vi "camara 2.1.vi"() -> ()   [LabVIEW 2010]
uses:
  <vilib>/addons/PixeLINK/Low Level Functions/CAMERA_FEATURES.llb/TDPU-CameraFeatures-PixelFormat.ctl
  <vilib>/addons/PixeLINK/Low Level Functions/ACQUISITION.llb/TDPU-Acquisition-StreamState.ctl
  <vilib>/addons/PixeLINK/Low Level Functions/CAMERA_FEATURES.llb/TDPU-CameraFeatures-FeatureFlags.ctl
  <vilib>/addons/PixeLINK/Low Level Functions/CAMERA_FEATURES.llb/TDPU-CameraFeatures-FeatureIds.ctl
panel:
  in  "Gain":dbl(slide) scale=0.0..25.0
  out "size(s)":i32
  out "Data OUT":u32[](array[numeric]) format="%x"
  out "Image":T1(plugin-control)
  out "output array":u64[][](array[numeric]) format="%x"
  in  "Exposure Time (ms)":dbl(slide) scale=0.1..2000.0
  in  "Streeam":bool
  in  "Pixel Format Requerido":T2 items=["PIXEL_FORMAT_MONO8", "PIXEL_FORMAT_MONO16", "PIXEL_FORMAT_YUV422", "PIXEL_FORMAT_BAYER8_GRBG", "PIXEL_FORMAT_BAYER16_GRBG", "PIXEL_FORMAT_RGB24", "PIXEL_FORMAT_RGB48", "PIXEL_FORMAT_BAYER8_RGGB", "PIXEL_FORMAT_BAYER8_GBRG ", "PIXEL_FORMAT_BAYER8_BGGR ", "PIXEL_FORMAT_BAYER16_RGGB ", "PIXEL_FORMAT_BAYER16_GBRG", "PIXEL_FORMAT_BAYER16_BGGR", "PIXEL_FORMAT_RGB32"]
  out "Numeric":i32
  in  "Stop App":bool
  out "Numero de Camaras":u32
  in  "Selector":u16(ring) items=["776002034"]
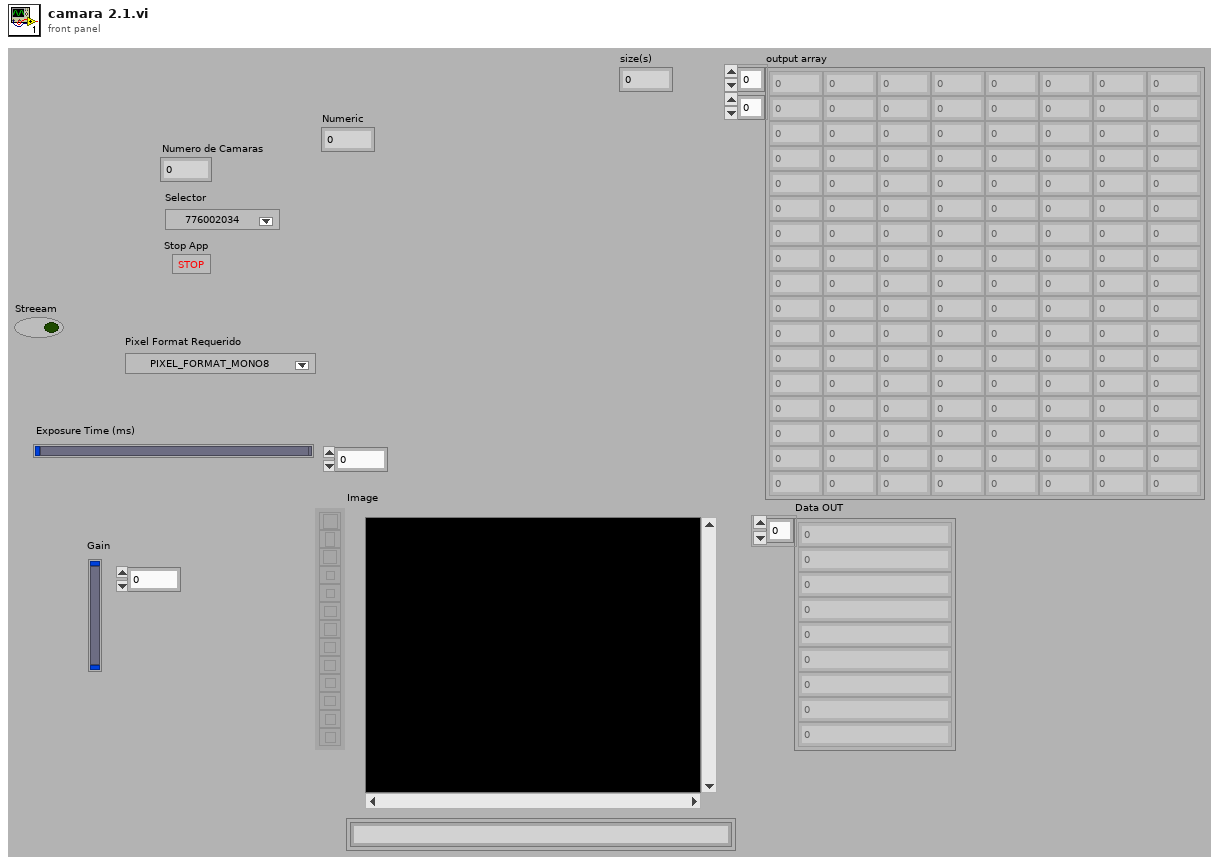
[diagram p1: front panel]
types:
  T1 = typedef "IMAQ Image.ctl" = refnum<image>
  T2 = typedef "TDPU-CameraFeatures-PixelFormat.ctl" = u16
  T3 = typedef "Image Type" = u32
  T4 = typedef "TDPU-Acquisition-StreamState.ctl" = u32
  T5 = typedef "TDPU-CameraFeatures-FeatureIds.ctl" = u32
  T6 = typedef "TDPU-CameraFeatures-FeatureFlags.ctl" = u32
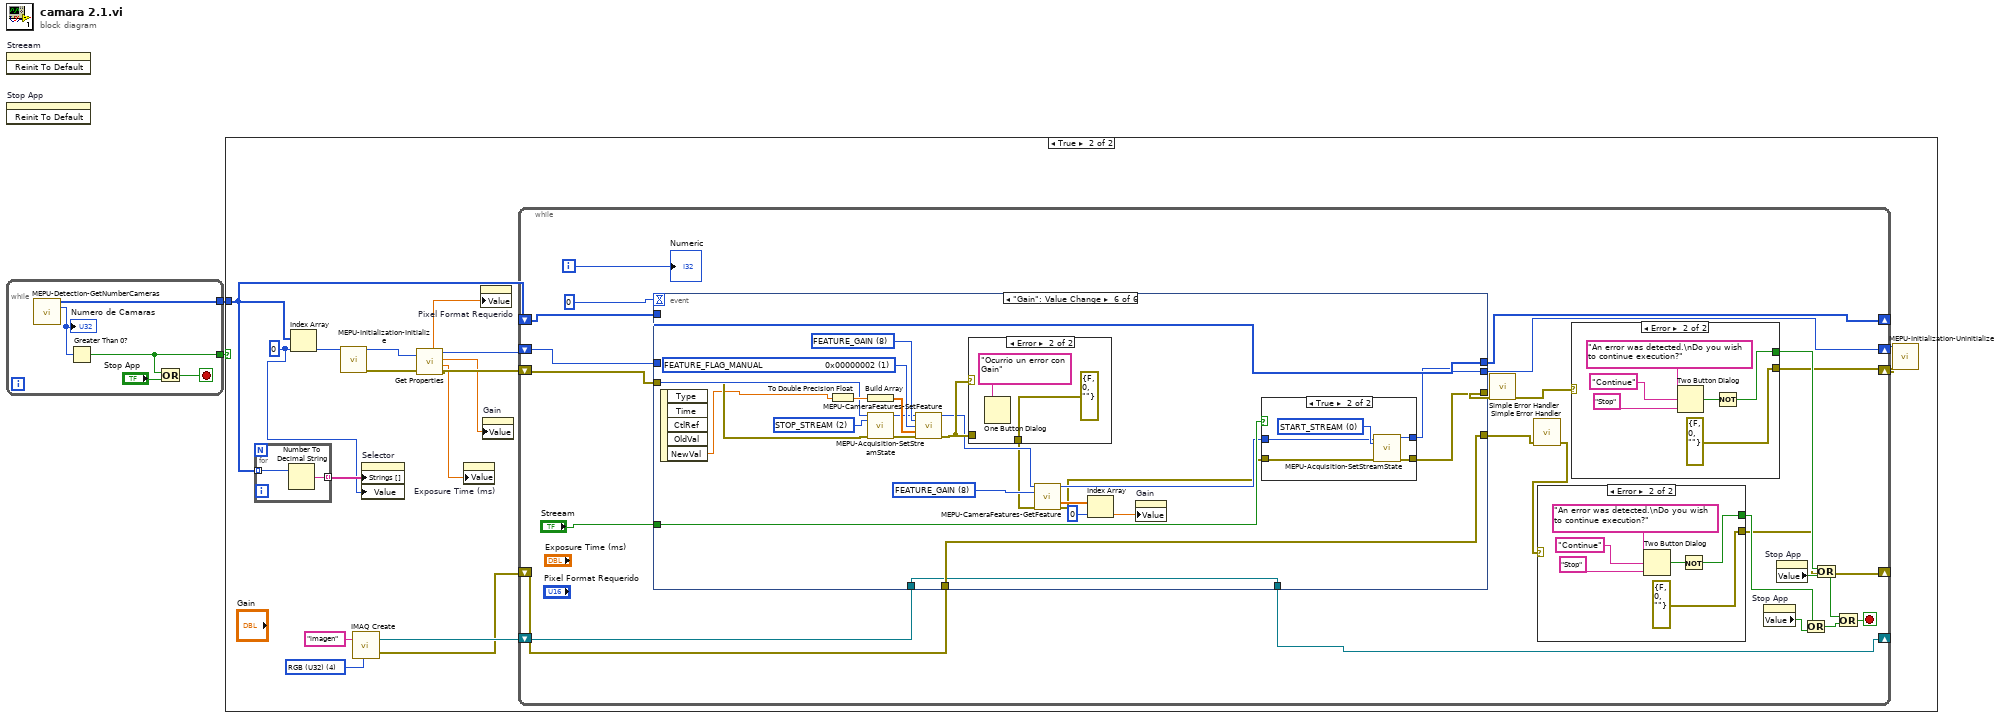
[diagram p0: block diagram]
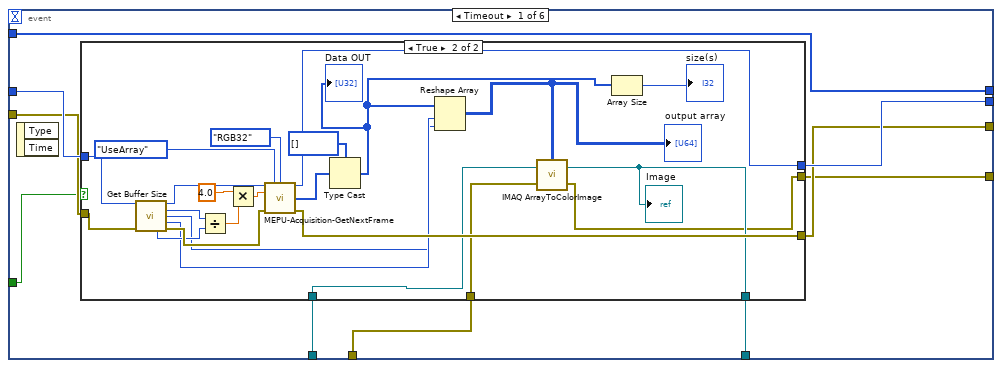
[diagram p5: hidden frame]
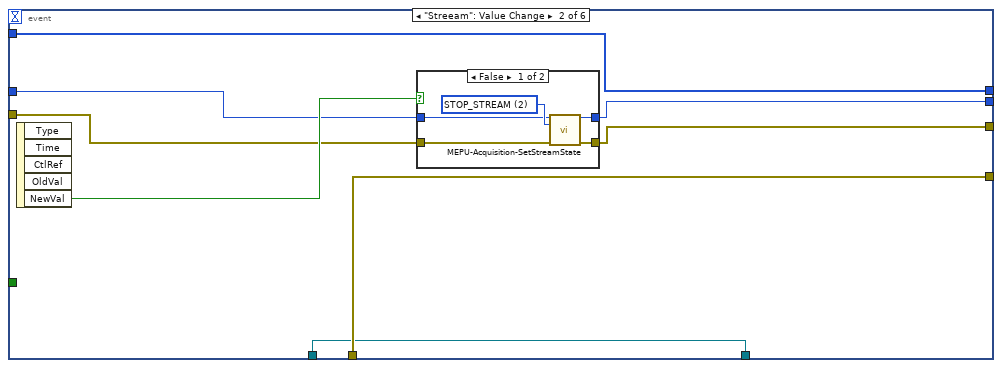
[diagram p7: hidden frame]
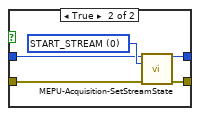
[diagram p8: hidden frame]
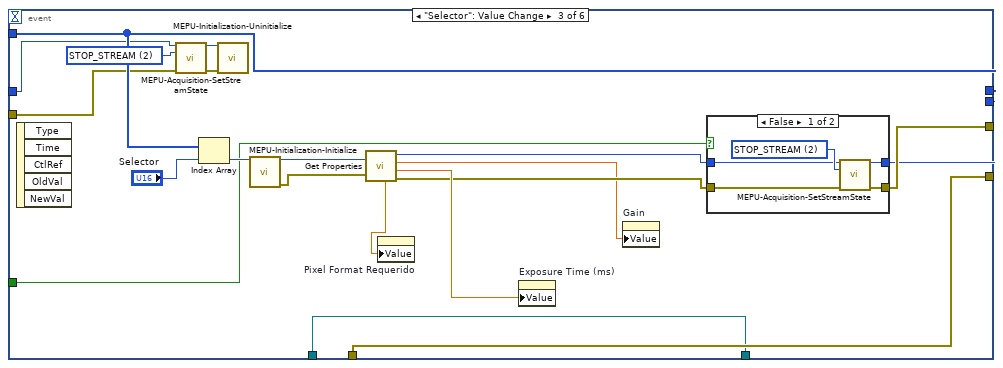
[diagram p9: hidden frame]
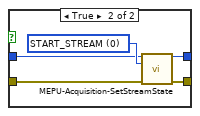
[diagram p10: hidden frame]
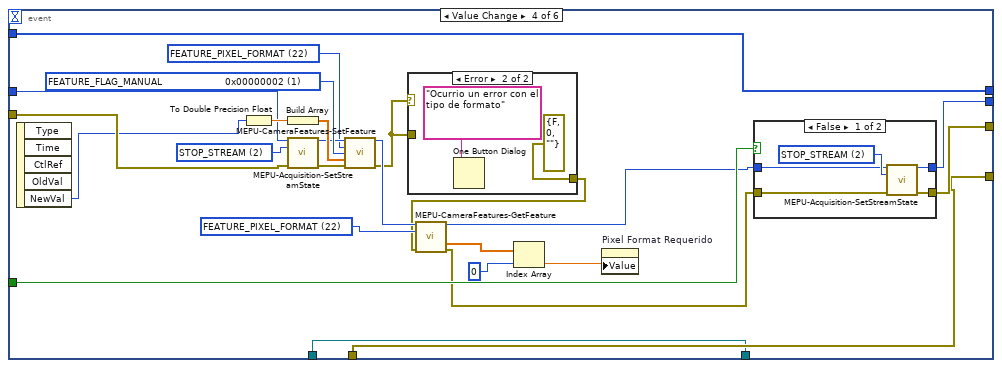
[diagram p11: hidden frame]
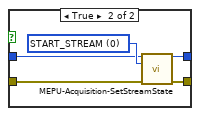
[diagram p12: hidden frame]
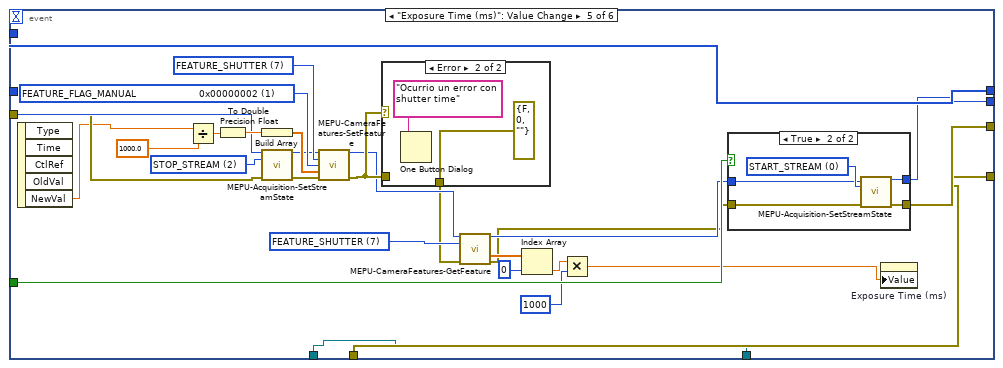
[diagram p14: hidden frame]
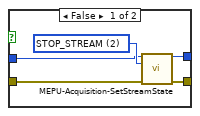
[diagram p15: hidden frame]
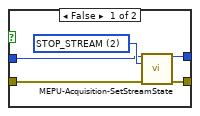
[diagram p17: hidden frame]
diagram:
  n1 = invoke on="Streeam" class="Bool (strict)" method="Reinit To Default"() -> ()  [unwired: 3 in, 3 out]
  n2 = invoke on="Stop App" class="Bool (strict)" method="Reinit To Default"() -> ()  [unwired: 3 in, 3 out]
  n3 = while {
    tunnel: [w7] -> w2
    tunnel: [w3] -> w1
    stop <- w5 stop-if-true
    n4 = call <vilib>:"MEPU-Detection-GetNumberCameras.vi"() -> ("LV_SerialNumbers OUT"=w7:u32[], "LV_NumberSerial OUT"=w4:u32)  [unwired: 13 in, 1 out]
    "Numero de Camaras" <- w4
    n5 = Greater Than 0?(x=w4) -> (x > 0?=w3:bool)
    n6 = Or(x=w3, y="Stop App") -> (x .or. y?=w5:bool)
  }
  n7 = case shown="True" w1 {
    tunnel: w2 -> [_ w21]
    frame False {
    }
    frame True {
      w15 = T3 4 items=["Grayscale (U8)", "Grayscale (I16)", "Grayscale (SGL)", "Complex (CSG)", "RGB (U32)", "HSL (U32)", "RGB (U64)", "Grayscale (U16)"] ("Image Type")
      w20 = 0
      n8 = for {
        tunnel: w21 -> [w269] mode=indexing
        tunnel: [w268] -> w23 mode=indexing
        n9 = Number To Decimal String(number=w269) -> (decimal integer string=w268:string)  [unwired: 1 in]
      }
      n10 = Index Array(array=w21, index=w20) -> (element=w22:u32)
      n11 = call <vilib>:"MEPU-Initialization-Initialize.vi"("uSerialNumber IN"=w22) -> ("phCamera OUT"=w14:u32, "Error OUT"=w13:errorcluster)  [unwired: 12 in, 1 out]
      n12 = call "IMAQ Create"("Image Name"="imagen", "Image Type"=w15) -> ("New Image"=w18:T1, "error out"=w16:errorcluster)  [unwired: 3 in]
      n13 = property on="Selector" class="Ring (strict)"("Strings []"=w23, "Value"=w20) -> ()  [unwired: 2 in, 2 out]
      n14 = call "Get Properties.vi"("phCamera IN"=w14, "Error IN"=w13) -> ("hCamera OUT"=w12:u32, "Gain OUT"=w10:dbl, "Shutter Time OUT (ms)"=w8:dbl, "Error OUT"=w11:errorcluster, "Pixel Format OUT"=w9:dbl)
      n15 = property on="Exposure Time (ms)" class="Slide (strict)"("Value"=w8) -> ()  [unwired: 2 in, 2 out]
      n16 = property on="Pixel Format Requerido" class="Ring (strict)"("Value"=w9) -> ()  [unwired: 2 in, 2 out]
      n17 = property on="Gain" class="Slide (strict)"("Value"=w10) -> ()  [unwired: 2 in, 2 out]
      n18 = while {
        shift-right: [w46] -> _
        shift-left: w21 -> [w47]
        shift-right: [w36] -> w19
        shift-left: w12 -> [w45]
        shift-right: [w41] -> _
        shift-left: w11 -> [w44]
        shift-right: [w26] -> _
        shift-left: w16 -> [w25]
        shift-right: [w24] -> _
        shift-left: w18 -> [w34]
        i -> [w40]
        stop <- w28 stop-if-true
        n19 = event shown="[5] \"Gain\": Value Change" {
          selector: _ -> [_ _ _ _ _ _]
          dyn-events: _ -> [_ _ _ _ _ _]
          timeout: 0 -> [_ _ _ _ _ _]
          tunnel: w47 -> [w73 w102 w137 w166 w208 w246]
          tunnel: [w71 w106 w128 w165 w207 w245] -> w36
          tunnel: [w68 w105 w129 w164 w206 w244] -> w37
          tunnel: [w73 w102 w137 w166 w208 w246] -> w46
          tunnel: w45 -> [w72 w108 w130 w171 w205 w243]
          tunnel: w44 -> [w70 w107 w131 w170 w204 w242]
          tunnel: "Streeam" -> [w69 _ w127 w163 w203 w241]
          tunnel: w34 -> [w67 w103 w125 w151 w189 w232]
          tunnel: w25 -> [w66 w104 w126 w162 w200 w240]
          tunnel: [w65 w104 w126 w162 w200 w240] -> w33
          tunnel: [w64 w103 w125 w151 w189 w232] -> w24
          event Timeout {
            n20 = event-data() -> ()  [unwired: 1 in, 2 out]
            n21 = case shown="True" w69 {
              tunnel: w72 -> [w77 w98]
              tunnel: [w76 w97] -> w68
              tunnel: [w77 w89] -> w71
              tunnel: w70 -> [w76 w96]
              tunnel: w67 -> [w74 w88]
              tunnel: w66 -> [w75 w87]
              tunnel: [w75 w78] -> w65
              tunnel: [w74 w86] -> w64
              frame False {
              }
              frame True {
                n22 = call "Get Buffer Size.vi"("phCamera IN"=w98, "Error IN"=w96) -> ("phCamera OUT"=w99:u32, "uBufferSize OUT"=w91:u32, "uWidth OUT"=w81:u32, "uHeight OUT"=w82:u32, "uBytesPerPixel OUT"=w90:u32, "Error OUT"=w101:errorcluster)  [unwired: 8 out]
                n23 = Divide(x=w91, y=w90) -> (x/y=w93:dbl)
                n24 = Multiply(x=4.0, y=w93) -> (x*y=w94:dbl)
                n25 = call <vilib>:"MEPU-Acquisition-GetNextFrame.vi"("hCamera IN"=w99, "Mode IN"=enum16{"UseArray", "UsePointer"}."UseArray", "OutputMode IN"=enum16{"Default", "RGB24", "RGB32"}."RGB32", "uBufferSize IN"=w94, "Error IN"=w101) -> ("hCamera OUT"=w89:u32, "Data OUT"=w80:u8[], "Error OUT"=w97:errorcluster)  [unwired: 6 in, 2 out]
                n26 = Type Cast(type=u32[] [] ("Data OUT"), x=w80) -> (*(type *) &x=w79:u32[])
                "Data OUT" <- w79
                n27 = Reshape Array(w79, w82, w81) -> (w85:u32[][])
                "output array" <- w85
                n28 = call "IMAQ ArrayToColorImage"("Image Pixels (U32)"=w85, "Image"=w88, "error in (no error)"=w87) -> ("Image Out"=w86:T1, "error out"=w78:errorcluster)  [unwired: 2 in]
                "Image" <- w86
                n29 = Array Size(array=w79) -> (size(s)=→"size(s)":i32)
              }
            }
          }
          event "Streeam": Value Change {
            n30 = event-data() -> ("NewVal"=w109:bool)  [unwired: 1 in, 4 out]
            n31 = case shown="False" w109 {
              tunnel: w108 -> [w113 w118]
              tunnel: w107 -> [w112 w117]
              tunnel: [w110 w116] -> w105
              tunnel: [w111 w115] -> w106
              frame False {
                w114 = T4 2 items=["START_STREAM", "PAUSE_STREAM", "STOP_STREAM"] ("uStreamState IN")
                n32 = call <vilib>:"MEPU-Acquisition-SetStreamState.vi"("hCamera IN"=w113, "uStreamState IN"=w114, "Error IN"=w112) -> ("hCamera OUT"=w111:u32, "Error OUT"=w110:errorcluster)  [unwired: 11 in]
              }
              frame True {
                w119 = T4 0 items=["START_STREAM", "PAUSE_STREAM", "STOP_STREAM"] ("uStreamState IN")
                n33 = call <vilib>:"MEPU-Acquisition-SetStreamState.vi"("hCamera IN"=w118, "uStreamState IN"=w119, "Error IN"=w117) -> ("hCamera OUT"=w115:u32, "Error OUT"=w116:errorcluster)  [unwired: 11 in]
              }
            }
          }
          event "Selector": Value Change {
            w134 = T4 2 items=["START_STREAM", "PAUSE_STREAM", "STOP_STREAM"] ("uStreamState IN")
            n34 = event-data() -> ()  [unwired: 1 in, 5 out]
            n35 = call <vilib>:"MEPU-Acquisition-SetStreamState.vi"("hCamera IN"=w130, "uStreamState IN"=w134, "Error IN"=w131) -> ("hCamera OUT"=w132:u32, "Error OUT"=w133:errorcluster)  [unwired: 11 in]
            n36 = Index Array(array=w137, index="Selector") -> (element=w138:u32)
            n37 = call <vilib>:"MEPU-Initialization-Uninitialize.vi"("hCamera IN"=w132, "Error IN"=w133) -> ()  [unwired: 13 in, 1 out]
            n38 = call <vilib>:"MEPU-Initialization-Initialize.vi"("uSerialNumber IN"=w138) -> ("phCamera OUT"=w136:u32, "Error OUT"=w135:errorcluster)  [unwired: 12 in, 1 out]
            n39 = call "Get Properties.vi"("phCamera IN"=w136, "Error IN"=w135) -> ("hCamera OUT"=w121:u32, "Gain OUT"=w120:dbl, "Shutter Time OUT (ms)"=w123:dbl, "Error OUT"=w122:errorcluster, "Pixel Format OUT"=w124:dbl)
            n40 = property on="Pixel Format Requerido" class="Ring (strict)"("Value"=w124) -> ()  [unwired: 2 in, 2 out]
            n41 = property on="Exposure Time (ms)" class="Slide (strict)"("Value"=w123) -> ()  [unwired: 2 in, 2 out]
            n42 = property on="Gain" class="Slide (strict)"("Value"=w120) -> ()  [unwired: 2 in, 2 out]
            n43 = case shown="False" w127 {
              tunnel: w121 -> [w143 w148]
              tunnel: w122 -> [w142 w147]
              tunnel: [w140 w146] -> w129
              tunnel: [w141 w145] -> w128
              frame False {
                w144 = T4 2 items=["START_STREAM", "PAUSE_STREAM", "STOP_STREAM"] ("uStreamState IN")
                n44 = call <vilib>:"MEPU-Acquisition-SetStreamState.vi"("hCamera IN"=w143, "uStreamState IN"=w144, "Error IN"=w142) -> ("hCamera OUT"=w141:u32, "Error OUT"=w140:errorcluster)  [unwired: 11 in]
              }
              frame True {
                w149 = T4 0 items=["START_STREAM", "PAUSE_STREAM", "STOP_STREAM"] ("uStreamState IN")
                n45 = call <vilib>:"MEPU-Acquisition-SetStreamState.vi"("hCamera IN"=w148, "uStreamState IN"=w149, "Error IN"=w147) -> ("hCamera OUT"=w145:u32, "Error OUT"=w146:errorcluster)  [unwired: 11 in]
              }
            }
          }
          event Value Change {
            w156 = T5 22 items=["FEATURE_BRIGHTNESS", "FEATURE_EXPOSURE", "FEATURE_SHARPNESS", "FEATURE_WHITE_BAL", "FEATURE_HUE", "FEATURE_SATURATION", "FEATURE_GAMMA", "FEATURE_SHUTTER", "FEATURE_GAIN", "FEATURE_IRIS", "FEATURE_FOCUS", "FEATURE_TEMPERATURE", "FEATURE_TRIGGER", "FEATURE_ZOOM", "FEATURE_PAN", "FEATURE_TILT", "FEATURE_OPT_FILTER", "FEATURE_GPIO", "FEATURE_FRAME_RATE", "FEATURE_ROI", "FEATURE_FLIP", "FEATURE_PIXEL_ADDRESSING", "FEATURE_PIXEL_FORMAT", "FEATURE_EXTENDED_SHUTTER", "FEATURE_AUTO_ROI", "FEATURE_LOOKUP_TABLE", "FEATURE_MEMORY_CHANNEL", "FEATURE_WHITE_SHADING", "FEATURE_ROTATE", "FEATURE_IMAGER_CLK_DIVISOR", "FEATURE_TRIG_WITH_CNTRLD_LIGHT", "FEATURE_MAX_PIXEL_SIZE"] ("uFeatureId IN")
            w167 = T4 2 items=["START_STREAM", "PAUSE_STREAM", "STOP_STREAM"] ("uStreamState IN")
            w174 = T6 1 items=["FEATURE_FLAG_PRESENCE                 0x00000001", "FEATURE_FLAG_MANUAL                     0x00000002", "FEATURE_FLAG_AUTO                         0x00000004", "FEATURE_FLAG_ONEPUSH                   0x00000008", "FEATURE_FLAG_OFF                            0x00000010", "FEATURE_FLAG_DESC_SUPPORTED    0x00000020", "FEATURE_FLAG_READ_ONLY               0x00000040"] ("uFlags IN")
            w161 = T5 22 items=["FEATURE_BRIGHTNESS", "FEATURE_EXPOSURE", "FEATURE_SHARPNESS", "FEATURE_WHITE_BAL", "FEATURE_HUE", "FEATURE_SATURATION", "FEATURE_GAMMA", "FEATURE_SHUTTER", "FEATURE_GAIN", "FEATURE_IRIS", "FEATURE_FOCUS", "FEATURE_TEMPERATURE", "FEATURE_TRIGGER", "FEATURE_ZOOM", "FEATURE_PAN", "FEATURE_TILT", "FEATURE_OPT_FILTER", "FEATURE_GPIO", "FEATURE_FRAME_RATE", "FEATURE_ROI", "FEATURE_FLIP", "FEATURE_PIXEL_ADDRESSING", "FEATURE_PIXEL_FORMAT", "FEATURE_EXTENDED_SHUTTER", "FEATURE_AUTO_ROI", "FEATURE_LOOKUP_TABLE", "FEATURE_MEMORY_CHANNEL", "FEATURE_WHITE_SHADING", "FEATURE_ROTATE", "FEATURE_IMAGER_CLK_DIVISOR", "FEATURE_TRIG_WITH_CNTRLD_LIGHT", "FEATURE_MAX_PIXEL_SIZE"] ("uFeatureId IN")
            n46 = event-data() -> ("NewVal"=w152:T2)  [unwired: 1 in, 4 out]
            n47 = To Double Precision Float(number=w152) -> (double precision float=w172:dbl)
            n48 = Build Array(w172) -> (w173:dbl[])
            n49 = call <vilib>:"MEPU-Acquisition-SetStreamState.vi"("hCamera IN"=w171, "uStreamState IN"=w167, "Error IN"=w170) -> ("hCamera OUT"=w169:u32, "Error OUT"=w168:errorcluster)  [unwired: 11 in]
            n50 = call <vilib>:"MEPU-CameraFeatures-SetFeature.vi"("hCamera IN"=w169, "uFeatureId IN"=w161, "uFlags IN"=w174, "pParms IN"=w173, "Error IN"=w168) -> ("hCamera OUT"=w158:u32, "Error OUT"=w154:errorcluster)  [unwired: 8 in, 1 out]
            n51 = case shown="Error" w154 {
              tunnel: [w185 errorcluster {"status"=FALSE, "code"=0, "source"=""} ("Error OUT")] -> w153
              tunnel: w154 -> [w185 _]
              frame No Error {
              }
              frame Error {
                n52 = One Button Dialog(message="Ocurrio un error con el tipo de formato") -> ()  [unwired: 1 in, 1 out]
              }
            }
            n53 = call <vilib>:"MEPU-CameraFeatures-GetFeature.vi"("hCamera IN"=w158, "uFeatureId IN"=w156, "Error IN"=w153) -> ("hCamera OUT"=w157:u32, "pParms OUT"=w155:dbl[], "Error OUT"=w159:errorcluster)  [unwired: 8 in, 2 out]
            n54 = Index Array(array=w155, index=0) -> (element=w150:dbl)
            n55 = property on="Pixel Format Requerido" class="Ring (strict)"("Value"=w150) -> ()  [unwired: 2 in, 2 out]
            n56 = case shown="False" w163 {
              tunnel: w157 -> [w178 w183]
              tunnel: w159 -> [w177 w182]
              tunnel: [w175 w181] -> w164
              tunnel: [w176 w180] -> w165
              frame False {
                w179 = T4 2 items=["START_STREAM", "PAUSE_STREAM", "STOP_STREAM"] ("uStreamState IN")
                n57 = call <vilib>:"MEPU-Acquisition-SetStreamState.vi"("hCamera IN"=w178, "uStreamState IN"=w179, "Error IN"=w177) -> ("hCamera OUT"=w176:u32, "Error OUT"=w175:errorcluster)  [unwired: 11 in]
              }
              frame True {
                w184 = T4 0 items=["START_STREAM", "PAUSE_STREAM", "STOP_STREAM"] ("uStreamState IN")
                n58 = call <vilib>:"MEPU-Acquisition-SetStreamState.vi"("hCamera IN"=w183, "uStreamState IN"=w184, "Error IN"=w182) -> ("hCamera OUT"=w180:u32, "Error OUT"=w181:errorcluster)  [unwired: 11 in]
              }
            }
          }
          event "Exposure Time (ms)": Value Change {
            w195 = T5 7 items=["FEATURE_BRIGHTNESS", "FEATURE_EXPOSURE", "FEATURE_SHARPNESS", "FEATURE_WHITE_BAL", "FEATURE_HUE", "FEATURE_SATURATION", "FEATURE_GAMMA", "FEATURE_SHUTTER", "FEATURE_GAIN", "FEATURE_IRIS", "FEATURE_FOCUS", "FEATURE_TEMPERATURE", "FEATURE_TRIGGER", "FEATURE_ZOOM", "FEATURE_PAN", "FEATURE_TILT", "FEATURE_OPT_FILTER", "FEATURE_GPIO", "FEATURE_FRAME_RATE", "FEATURE_ROI", "FEATURE_FLIP", "FEATURE_PIXEL_ADDRESSING", "FEATURE_PIXEL_FORMAT", "FEATURE_EXTENDED_SHUTTER", "FEATURE_AUTO_ROI", "FEATURE_LOOKUP_TABLE", "FEATURE_MEMORY_CHANNEL", "FEATURE_WHITE_SHADING", "FEATURE_ROTATE", "FEATURE_IMAGER_CLK_DIVISOR", "FEATURE_TRIG_WITH_CNTRLD_LIGHT", "FEATURE_MAX_PIXEL_SIZE"] ("uFeatureId IN")
            w209 = T4 2 items=["START_STREAM", "PAUSE_STREAM", "STOP_STREAM"] ("uStreamState IN")
            w215 = T6 1 items=["FEATURE_FLAG_PRESENCE                 0x00000001", "FEATURE_FLAG_MANUAL                     0x00000002", "FEATURE_FLAG_AUTO                         0x00000004", "FEATURE_FLAG_ONEPUSH                   0x00000008", "FEATURE_FLAG_OFF                            0x00000010", "FEATURE_FLAG_DESC_SUPPORTED    0x00000020", "FEATURE_FLAG_READ_ONLY               0x00000040"] ("uFlags IN")
            w216 = T5 7 items=["FEATURE_BRIGHTNESS", "FEATURE_EXPOSURE", "FEATURE_SHARPNESS", "FEATURE_WHITE_BAL", "FEATURE_HUE", "FEATURE_SATURATION", "FEATURE_GAMMA", "FEATURE_SHUTTER", "FEATURE_GAIN", "FEATURE_IRIS", "FEATURE_FOCUS", "FEATURE_TEMPERATURE", "FEATURE_TRIGGER", "FEATURE_ZOOM", "FEATURE_PAN", "FEATURE_TILT", "FEATURE_OPT_FILTER", "FEATURE_GPIO", "FEATURE_FRAME_RATE", "FEATURE_ROI", "FEATURE_FLIP", "FEATURE_PIXEL_ADDRESSING", "FEATURE_PIXEL_FORMAT", "FEATURE_EXTENDED_SHUTTER", "FEATURE_AUTO_ROI", "FEATURE_LOOKUP_TABLE", "FEATURE_MEMORY_CHANNEL", "FEATURE_WHITE_SHADING", "FEATURE_ROTATE", "FEATURE_IMAGER_CLK_DIVISOR", "FEATURE_TRIG_WITH_CNTRLD_LIGHT", "FEATURE_MAX_PIXEL_SIZE"] ("uFeatureId IN")
            n59 = event-data() -> ("NewVal"=w190:dbl)  [unwired: 1 in, 4 out]
            n60 = Divide(x=w190, y=1000.0) -> (x/y=w202:dbl)
            n61 = To Double Precision Float(number=w202) -> (double precision float=w213:dbl)
            n62 = Build Array(w213) -> (w214:dbl[])
            n63 = call <vilib>:"MEPU-Acquisition-SetStreamState.vi"("hCamera IN"=w205, "uStreamState IN"=w209, "Error IN"=w204) -> ("hCamera OUT"=w211:u32, "Error OUT"=w210:errorcluster)  [unwired: 11 in]
            n64 = call <vilib>:"MEPU-CameraFeatures-SetFeature.vi"("hCamera IN"=w211, "uFeatureId IN"=w216, "uFlags IN"=w215, "pParms IN"=w214, "Error IN"=w210) -> ("hCamera OUT"=w194:u32, "Error OUT"=w212:errorcluster)  [unwired: 8 in, 1 out]
            n65 = case shown="Error" w212 {
              tunnel: [w227 errorcluster {"status"=FALSE, "code"=0, "source"=""} ("Error OUT")] -> w191
              tunnel: w212 -> [w227 _]
              frame No Error {
              }
              frame Error {
                n66 = One Button Dialog(message="Ocurrio un error con shutter time") -> ()  [unwired: 1 in, 1 out]
              }
            }
            n67 = call <vilib>:"MEPU-CameraFeatures-GetFeature.vi"("hCamera IN"=w194, "uFeatureId IN"=w195, "Error IN"=w191) -> ("hCamera OUT"=w193:u32, "pParms OUT"=w196:dbl[], "Error OUT"=w192:errorcluster)  [unwired: 8 in, 2 out]
            n68 = Index Array(array=w196, index=0) -> (element=w199:dbl)
            n69 = Multiply(x=w199, y=1000) -> (x*y=w188:dbl)
            n70 = case shown="True" w203 {
              tunnel: w192 -> [w220 w225]
              tunnel: [w218 w224] -> w206
              tunnel: [w219 w223] -> w207
              tunnel: w193 -> [w217 w222]
              frame False {
                w221 = T4 2 items=["START_STREAM", "PAUSE_STREAM", "STOP_STREAM"] ("uStreamState IN")
                n71 = call <vilib>:"MEPU-Acquisition-SetStreamState.vi"("hCamera IN"=w217, "uStreamState IN"=w221, "Error IN"=w220) -> ("hCamera OUT"=w219:u32, "Error OUT"=w218:errorcluster)  [unwired: 11 in]
              }
              frame True {
                w226 = T4 0 items=["START_STREAM", "PAUSE_STREAM", "STOP_STREAM"] ("uStreamState IN")
                n72 = call <vilib>:"MEPU-Acquisition-SetStreamState.vi"("hCamera IN"=w222, "uStreamState IN"=w226, "Error IN"=w225) -> ("hCamera OUT"=w223:u32, "Error OUT"=w224:errorcluster)  [unwired: 11 in]
              }
            }
            n73 = property on="Exposure Time (ms)" class="Slide (strict)"("Value"=w188) -> ()  [unwired: 2 in, 2 out]
          }
          event "Gain": Value Change {
            w237 = T5 8 items=["FEATURE_BRIGHTNESS", "FEATURE_EXPOSURE", "FEATURE_SHARPNESS", "FEATURE_WHITE_BAL", "FEATURE_HUE", "FEATURE_SATURATION", "FEATURE_GAMMA", "FEATURE_SHUTTER", "FEATURE_GAIN", "FEATURE_IRIS", "FEATURE_FOCUS", "FEATURE_TEMPERATURE", "FEATURE_TRIGGER", "FEATURE_ZOOM", "FEATURE_PAN", "FEATURE_TILT", "FEATURE_OPT_FILTER", "FEATURE_GPIO", "FEATURE_FRAME_RATE", "FEATURE_ROI", "FEATURE_FLIP", "FEATURE_PIXEL_ADDRESSING", "FEATURE_PIXEL_FORMAT", "FEATURE_EXTENDED_SHUTTER", "FEATURE_AUTO_ROI", "FEATURE_LOOKUP_TABLE", "FEATURE_MEMORY_CHANNEL", "FEATURE_WHITE_SHADING", "FEATURE_ROTATE", "FEATURE_IMAGER_CLK_DIVISOR", "FEATURE_TRIG_WITH_CNTRLD_LIGHT", "FEATURE_MAX_PIXEL_SIZE"] ("uFeatureId IN")
            w247 = T4 2 items=["START_STREAM", "PAUSE_STREAM", "STOP_STREAM"] ("uStreamState IN")
            w253 = T6 1 items=["FEATURE_FLAG_PRESENCE                 0x00000001", "FEATURE_FLAG_MANUAL                     0x00000002", "FEATURE_FLAG_AUTO                         0x00000004", "FEATURE_FLAG_ONEPUSH                   0x00000008", "FEATURE_FLAG_OFF                            0x00000010", "FEATURE_FLAG_DESC_SUPPORTED    0x00000020", "FEATURE_FLAG_READ_ONLY               0x00000040"] ("uFlags IN")
            w254 = T5 8 items=["FEATURE_BRIGHTNESS", "FEATURE_EXPOSURE", "FEATURE_SHARPNESS", "FEATURE_WHITE_BAL", "FEATURE_HUE", "FEATURE_SATURATION", "FEATURE_GAMMA", "FEATURE_SHUTTER", "FEATURE_GAIN", "FEATURE_IRIS", "FEATURE_FOCUS", "FEATURE_TEMPERATURE", "FEATURE_TRIGGER", "FEATURE_ZOOM", "FEATURE_PAN", "FEATURE_TILT", "FEATURE_OPT_FILTER", "FEATURE_GPIO", "FEATURE_FRAME_RATE", "FEATURE_ROI", "FEATURE_FLIP", "FEATURE_PIXEL_ADDRESSING", "FEATURE_PIXEL_FORMAT", "FEATURE_EXTENDED_SHUTTER", "FEATURE_AUTO_ROI", "FEATURE_LOOKUP_TABLE", "FEATURE_MEMORY_CHANNEL", "FEATURE_WHITE_SHADING", "FEATURE_ROTATE", "FEATURE_IMAGER_CLK_DIVISOR", "FEATURE_TRIG_WITH_CNTRLD_LIGHT", "FEATURE_MAX_PIXEL_SIZE"] ("uFeatureId IN")
            n74 = event-data() -> ("NewVal"=w231:dbl)  [unwired: 1 in, 4 out]
            n75 = To Double Precision Float(number=w231) -> (double precision float=w251:dbl)
            n76 = Build Array(w251) -> (w252:dbl[])
            n77 = call <vilib>:"MEPU-Acquisition-SetStreamState.vi"("hCamera IN"=w243, "uStreamState IN"=w247, "Error IN"=w242) -> ("hCamera OUT"=w249:u32, "Error OUT"=w248:errorcluster)  [unwired: 11 in]
            n78 = call <vilib>:"MEPU-CameraFeatures-SetFeature.vi"("hCamera IN"=w249, "uFeatureId IN"=w254, "uFlags IN"=w253, "pParms IN"=w252, "Error IN"=w248) -> ("hCamera OUT"=w236:u32, "Error OUT"=w250:errorcluster)  [unwired: 8 in, 1 out]
            n79 = case shown="Error" w250 {
              tunnel: [w265 errorcluster {"status"=FALSE, "code"=0, "source"=""} ("Error OUT")] -> w233
              tunnel: w250 -> [w265 _]
              frame No Error {
              }
              frame Error {
                n80 = One Button Dialog(message="Ocurrio un error con Gain") -> ()  [unwired: 1 in, 1 out]
              }
            }
            n81 = call <vilib>:"MEPU-CameraFeatures-GetFeature.vi"("hCamera IN"=w236, "uFeatureId IN"=w237, "Error IN"=w233) -> ("hCamera OUT"=w235:u32, "pParms OUT"=w238:dbl[], "Error OUT"=w234:errorcluster)  [unwired: 8 in, 2 out]
            n82 = Index Array(array=w238, index=0) -> (element=w230:dbl)
            n83 = property on="Gain" class="Slide (strict)"("Value"=w230) -> ()  [unwired: 2 in, 2 out]
            n84 = case shown="True" w241 {
              tunnel: w234 -> [w258 w263]
              tunnel: [w256 w262] -> w244
              tunnel: [w257 w261] -> w245
              tunnel: w235 -> [w255 w260]
              frame False {
                w259 = T4 2 items=["START_STREAM", "PAUSE_STREAM", "STOP_STREAM"] ("uStreamState IN")
                n85 = call <vilib>:"MEPU-Acquisition-SetStreamState.vi"("hCamera IN"=w255, "uStreamState IN"=w259, "Error IN"=w258) -> ("hCamera OUT"=w257:u32, "Error OUT"=w256:errorcluster)  [unwired: 11 in]
              }
              frame True {
                w264 = T4 0 items=["START_STREAM", "PAUSE_STREAM", "STOP_STREAM"] ("uStreamState IN")
                n86 = call <vilib>:"MEPU-Acquisition-SetStreamState.vi"("hCamera IN"=w260, "uStreamState IN"=w264, "Error IN"=w263) -> ("hCamera OUT"=w261:u32, "Error OUT"=w262:errorcluster)  [unwired: 11 in]
              }
            }
          }
        }
        n87 = call <vilib>:"Simple Error Handler.vi"("error in (no error)"=w37) -> ("error out"=w43:errorcluster)  [unwired: 1 in, 7 out]
        n88 = call <vilib>:"Simple Error Handler.vi"("error in (no error)"=w33) -> ("error out"=w32:errorcluster)  [unwired: 1 in, 7 out]
        n89 = case shown="Error" w32 {
          selector: w32 -> [w49 _]
          tunnel: [w49 errorcluster {"status"=FALSE, "code"=0, "source"=""} ("error IO")] -> w26
          tunnel: [FALSE ("T button?") w51] -> w27
          frame No Error {
          }
          frame Error {
            n90 = Two Button Dialog(message="An error was detected.\nDo you wish to continue execution?", 1:"Stop" ("F button name (\"Cancel\")"), 2:"Continue" ("T button name (\"OK\")")) -> (T button?=w52:bool)
            n91 = Not(x=w52) -> (.not. x?=w51:bool)
          }
        }
        n92 = case shown="Error" w43 {
          selector: w43 -> [w57 _]
          tunnel: [w57 errorcluster {"status"=FALSE, "code"=0, "source"=""} ("error IO")] -> w41
          tunnel: [FALSE ("T button?") w59] -> w42
          frame No Error {
          }
          frame Error {
            n93 = Two Button Dialog(message="An error was detected.\nDo you wish to continue execution?", 1:"Stop" ("F button name (\"Cancel\")"), 2:"Continue" ("T button name (\"OK\")")) -> (T button?=w60:bool)
            n94 = Not(x=w60) -> (.not. x?=w59:bool)
          }
        }
        n95 = property on="Stop App" class="Bool (strict)"() -> ("Value"=w31:bool)  [unwired: 2 in, 2 out]
        n96 = property on="Stop App" class="Bool (strict)"() -> ("Value"=w38:bool)  [unwired: 2 in, 2 out]
        n97 = Or(x=w27, y=w31) -> (x .or. y?=w29:bool)
        n98 = Or(x=w42, y=w38) -> (x .or. y?=w30:bool)
        n99 = Or(x=w30, y=w29) -> (x .or. y?=w28:bool)
        "Numeric" <- w40
      }
      n100 = call <vilib>:"MEPU-Initialization-Uninitialize.vi"("hCamera IN"=w19) -> ()  [unwired: 14 in, 1 out]
    }
  }
